vi "PH_Sequencer.set PP CurrentMeas Settings.vi"(0 "i ref in":refnum<vi>, 2 "linked?":T1 items=["undefined", "executing constructor", "_new: error", "_new: o.k.", "executing destructor"], 5 "error in (no error)":errorcluster) -> (14 "i ref out":refnum<vi>, 19 "error out":errorcluster)   [LabVIEW 2014, in "PH_Sequencer.lvlib"]
doc: "This VI gets whether the Current Measurement instance is alive or not."
uses:
  PH_Sequencer.lvlib
  CSCore/CSSystem/CSSystemLib/CSSystemLib.object condition.ctl
  PH_PP_CurrentMeas/PH_PP_CurrentMeas.lvlib
  CSCore/CSSystem/CSSystemLib/CSSystemLib.lvlib
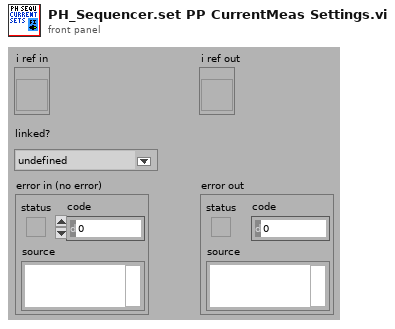
[diagram p1: front panel]
types:
  T1 = typedef "CSSystemLib.lvlib/CSSystemLib.object condition.ctl" = i32
  T2 = typedef "PH_Sequencer.lvlib/PH_Sequencer.i attribute.ctl" = cluster{"GUI Refs":cluster{"Main Off":refnum<vi>, "Fire":refnum<vi>, "Status":refnum<vi>, "Ready":refnum<vi>, "Waiting Time":refnum<vi>, "Timeout":refnum<vi>, "PPMA Ready":refnum<vi>, "Sequencer SM State":refnum<vi>, "PPPA Ready":refnum<vi>, "Calorimeter":refnum<vi>, "Beamline Ready":refnum<vi>, "Clear Beamline":refnum<vi>, "Linkage PPMA Rods":refnum<vi>, "Linkage Current PA":refnum<vi>, "Linkage Current MA":refnum<vi>, "Timing Ready":refnum<vi>, "State Timing":refnum<vi>, "Force Timing":refnum<vi>, "PSDB Shot Comment":refnum<vi>, "State PA Backreflection":refnum<vi>, "Beamline Z6 Ready":refnum<vi>, "Clear Z6 Beamline":refnum<vi>, "Sequence length":refnum<vi>, "Timing Mode":refnum<vi>, "Slow Trigger Settings":refnum<vi>, "Experiment Description":refnum<vi>, "State PSDB":refnum<vi>, "PSDB Ready":refnum<vi>, "Set PSDB Settings":refnum<vi>, "Get PSDB Info":refnum<vi>, "Take Snapshot":refnum<vi>, "Shottype":refnum<vi>, "Experiment":refnum<vi>, "Phase Frontends":refnum<vi>, "PP 45mm PILC in use":refnum<vi>}, "Status Info":cluster{"Machine Status":T3, "WaitingTime":i32, "Timeout":bool}, "Readyness":cluster{"Ready to shot":bool, "PPMA Ready":bool, "PPPA Ready":bool, "BL Ready":bool, "Timing Ready":bool, "BL Z6 Ready":bool, "PSDBReady":bool}, "Instancenames":cluster{"PPMA Rods":string, "PP Current Meas":string, "PH Beamline Chief":string, "PA Backrefl Meas":string, "Z6 Beamline Chief":string}, "Data to read":bool, "Calorimeter":cluster{"Instancename":string, "On":bool, "linked":bool}, "Linkage":cluster{"PPMA Rods":bool, "PP Current Meas":bool, "PHELIX Beamline Chief":bool, "PA Backrefl Meas":bool, "Z6 Beamline Chief":bool}, "Timing":cluster{"Instance":string, "linked":bool, "Status":T3, "Timing Mode":T4, "Slow Trigger Settings":T5, "Info available":cluster{"ext SlowTrigger":bool, "T2":bool, "Mode":bool, "Delay Slow Trigger":bool, "Phase FEs":bool}, "FE Phase":T6}, "Service ID R2S":i32, "PSDB":cluster{"Controller Instance":string, "Controller Status":T3, "Controller linked":bool, "Settings acknowledged":bool, "Current Experiment ID":i16, "Current Shot Type":i16, "Current Comment":string, "Remember Settings":bool, "Write 2 early":bool}, "PSDB Data":cluster{"Main Off?":bool, "Sequence Length":dbl, "Sequence startet":timestamp}, "6P 4Q Positions":cluster{"Instancename":string, "linked":bool, "Position":T7}[], "PUs":T8[]}
  T3 = typedef "PH_StatusHandler.lvlib/PH_StatusHandler.Status.ctl" = i16
  T4 = typedef "PH_Timing.lvlib/PH_Timing.Timing Mode.ctl" = cluster{"T2":i16, "Modeselector":enum32{"10 Hz", "0.5 Hz", "Shot"}}
  T5 = typedef "PH_Timing.lvlib/PH_Timing.Slow Trigger Settings.ctl" = cluster{"Delay":dbl, "externally triggered?":bool}
  T6 = typedef "PH_Timing.lvlib/PH_Timing.Phase FEs.ctl" = cluster{"Phase":dbl}
  T7 = typedef "PH_4_Pos_Selector.lvlib/PH_4_Pos_Selector.Position Selector.ctl" = u16
  T8 = typedef "PH_Sequencer.lvlib/PH_Sequencer.Head.ctl" = cluster{"PowerUnit":T9, "GUI Ref":refnum<vi>, "Information":T10, "linked?":bool, "GUI Ref Current Voltage":refnum<vi>}
  T9 = typedef "PH_PP_Common.lvlib/PH_PP_Common.PUs.ctl" = enum16{"no Info", "PA-19mm-1", "PA-19mm-2", "PA-45mm-PILC", "PA-45mm-MAIN", "MA-PU-1", "MA-PU-2", "MA-PU-3", "MA-PU-4", "MA-PU-5", "MA-PU-6", "MA-FR", "MA-PILC", "PA-45mm-DP"}
  T10 = typedef "PH_Sequencer.lvlib/PH_Sequencer.PU Information.ctl" = cluster{"State":T3, "Waiting Time [s]":dbl, "PU State SM":T11, "PU Timeout SM":T11}
  T11 = typedef "PH_PowerUnit_BaseClass.lvlib/PH_PowerUnit_BaseClass.SM States.ctl" = enum16{".", "Stand by", "Switch PU on", "Configure", "Set Default Voltage", "Set STANDBY", "Set READY", "Wait for Shot Cmd", "Open Dump Rods", "Open Ross Relais", "Close Ross Relais", "Switch PSU on", "Switch PSU off", "Charge", "Switch GD Channel on", "Close Dump Rods", "Rods-TO", "RR-TO", "PSU-TO", "Trigger-TO"}
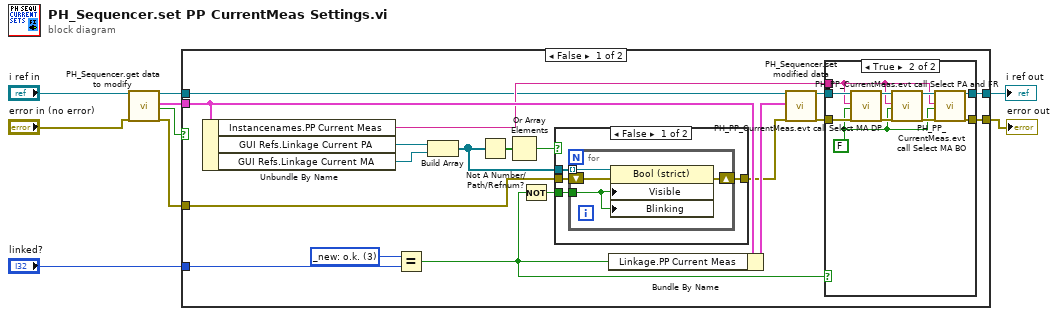
[diagram p0: block diagram]
diagram:
  n1 = call "PH_Sequencer.get data to modify.vi"("i ref in"="i ref in", "error in (no error)"="error in (no error)") -> ("i ref out"=w7:refnum<vi>, "i attribute"=w9:T2, "timed out"=w4:bool, "error out"=w5:errorcluster)  [unwired: 14 in]
  n2 = case shown="False" w4 {
    tunnel: w7 -> [w22 w51]
    tunnel: [w11 w51] -> w2
    tunnel: w5 -> [w12 w50]
    tunnel: [w10 w50] -> w1
    tunnel: w9 -> [w28 _]
    tunnel: "linked?" -> [w13 _]
    frame False {
      w15 = T1 3 items=["undefined", "executing constructor", "_new: error", "_new: o.k.", "executing destructor"] ("x")
      n3 = Unbundle By Name(w28) -> ("Instancenames.PP Current Meas"=w23:string, "GUI Refs.Linkage Current PA"=w18:refnum<vi>, "GUI Refs.Linkage Current MA"=w21:refnum<vi>)
      n4 = Equal?(x=w15, y=w13) -> (x = y?=w14:bool)
      n5 = Build Array(w18, w21) -> (w17:refnum<vi>[])
      n6 = Not A Number/Path/Refnum?(number/path/refnum=w17) -> (NaN/Path/Refnum?=w20:bool[])
      n7 = Or Array Elements(Boolean array=w20) -> (logical OR=w19:bool)
      n8 = Not(x=w14) -> (.not. x?=w16:bool)
      n9 = case shown="False" w19 {
        tunnel: w17 -> [w44 _]
        tunnel: w12 -> [w43 w49]
        tunnel: [w42 w49] -> w26
        tunnel: w16 -> [w41 _]
        frame False {
          n10 = for {
            tunnel: w44 -> [w48] mode=indexing
            tunnel: w41 -> [w45]
            shift-right: [w46] -> w42
            shift-left: w43 -> [w47]
            n11 = property class="Bool (strict)"(reference=w48, error in=w47, "Visible"=w45, "Blinking"=w45) -> (error out=w46:errorcluster)  [unwired: 1 out]
          }
        }
        frame True {
        }
      }
      n12 = Bundle By Name(cluster=w28, "Linkage.PP Current Meas"=w14) -> (w27:T2)
      n13 = call "PH_Sequencer.set modified data.vi"("i ref in"=w22, "i attribute"=w27, "error in (no error)"=w26) -> ("i ref out"=w25:refnum<vi>, "error out"=w24:errorcluster)  [unwired: 15 in]
      n14 = case shown="True" w14 {
        tunnel: w25 -> [w30 w37]
        tunnel: [w30 w35] -> w11
        tunnel: w24 -> [w29 w38]
        tunnel: [w29 w33] -> w10
        tunnel: w23 -> [_ w32]
        frame False {
        }
        frame True {
          w31 = FALSE
          n15 = call "PH_PP_CurrentMeas.evt call Select MA DP.vi"("i ref in"=w37, "Instance name"=w32, "Select MA DP"=w31, "error in (no error)"=w38) -> ("i ref out"=w40:refnum<vi>, "error out"=w39:errorcluster)  [unwired: 14 in]
          n16 = call "PH_PP_CurrentMeas.evt call Select PA and FR.vi"("i ref in"=w40, "Instance name"=w32, "Select PA/FR"=w31, "error in (no error)"=w39) -> ("i ref out"=w36:refnum<vi>, "error out"=w34:errorcluster)  [unwired: 14 in]
          n17 = call "PH_PP_CurrentMeas.evt call Select MA BO.vi"("i ref in"=w36, "Instance name"=w32, "Select MA BO"=w31, "error in (no error)"=w34) -> ("i ref out"=w35:refnum<vi>, "error out"=w33:errorcluster)  [unwired: 14 in]
        }
      }
    }
    frame True {
    }
  }
  "i ref out" <- w2
  "error out" <- w1
